vi "TDC_Selection.vi"(11 "TDC#":T1(ring)) -> (3 "TDC":sgl)   [LabVIEW 2015, in "ECS-RT.lvlib"]
uses:
  ECS-RT.lvlib
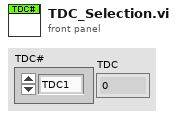
[diagram p1: front panel]
types:
  T1 = enum32{"TDC1", "TDC2", "TDC3", "TDC4", "TDC5", "TDC6", "TDC7", "TDC8"}
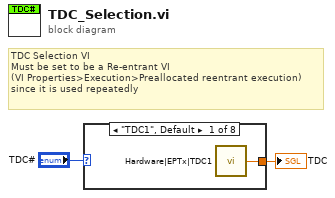
[diagram p0: block diagram]
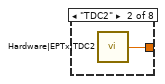
[diagram p2: hidden frame]
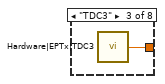
[diagram p3: hidden frame]
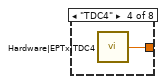
[diagram p4: hidden frame]
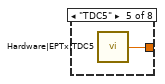
[diagram p5: hidden frame]
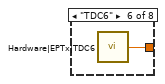
[diagram p6: hidden frame]
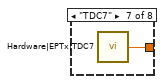
[diagram p7: hidden frame]
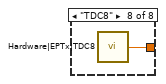
[diagram p8: hidden frame]
diagram:
  # "TDC Selection VI\nMust be set to be a Re-entrant VI \n(VI Properties>Execution>Preallocated reentrant execution)\nsince it is used repeatedly"
  n1 = case shown="\"TDC1\", Default" "TDC#" {
    tunnel: [w3 w4 w5 w6 w7 w8 w9 w10] -> w1
    frame "TDC1", Default {
      n2 = call "Hardware|EPTx|TDC1"() -> ("Value"=w3:sgl)
    }
    frame "TDC2" {
      n3 = call "Hardware|EPTx|TDC2"() -> ("Value"=w4:sgl)
    }
    frame "TDC3" {
      n4 = call "Hardware|EPTx|TDC3"() -> ("Value"=w5:sgl)
    }
    frame "TDC4" {
      n5 = call "Hardware|EPTx|TDC4"() -> ("Value"=w6:sgl)
    }
    frame "TDC5" {
      n6 = call "Hardware|EPTx|TDC5"() -> ("Value"=w7:sgl)
    }
    frame "TDC6" {
      n7 = call "Hardware|EPTx|TDC6"() -> ("Value"=w8:sgl)
    }
    frame "TDC7" {
      n8 = call "Hardware|EPTx|TDC7"() -> ("Value"=w9:sgl)
    }
    frame "TDC8" {
      n9 = call "Hardware|EPTx|TDC8"() -> ("Value"=w10:sgl)
    }
  }
  "TDC" <- w1
